vi "GetContextHelpInfo.vi"(0 "reference in":refnum<class "DQMHModuleNode.lvclass">, 1 "MousePos":T1 {"y" format="%.2f"; "x" format="%.2f"}, 5 "error in (no error)":errorcluster) -> (14 "reference out":refnum<class "DQMHModuleNode.lvclass">, 15 "ContextHelpInfoExist":bool, 16 "ContextHelpInfo":variant, 19 "error out":errorcluster)   [LabVIEW 2014, in "DQMHModuleNode.lvclass"]
doc: "GetContextHelpInfo"
uses:
  <resource>/Framework/Providers/Open_GDS/UML/DQMHModuleNode_class/DQMHModuleNode.lvclass
  <resource>/Framework/Providers/Open_GDS/UML/General/Point/Point Point2D.ctl
  <resource>/Framework/Providers/Open_GDS/UML/MultiLineString_class/MultiLineString.lvclass
  <resource>/Framework/Providers/Open_GDS/ClassProviders/Provider_BaseClassInterface/ClassReader_class/ClassReader.lvclass
  <resource>/Framework/Providers/Open_GDS/UML/RectangularNode_class/RectangularNode.lvclass
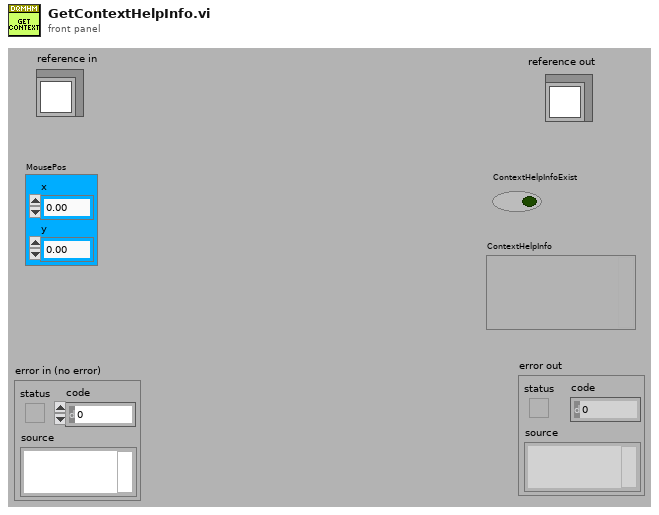
[diagram p1: front panel]
types:
  T1 = typedef "Point Point2D.ctl" = cluster{"x":dbl, "y":dbl}
  T2 = typedef "DQMHModuleNode.lvclass/ObjectAttributes.ctl" = cluster{"midHeight":dbl, "botHeight":dbl, "Name":refnum<class "MultiLineString.lvclass">, "Description":refnum<class "MultiLineString.lvclass">, "InternalData":refnum<class "MultiLineString.lvclass">, "Events":refnum<class "MultiLineString.lvclass">, "DEFAULT_COMPARTMENT_HEIGHT":i32, "DEFAULT_WIDTH":i32, "DEFAULT_HEIGHT":i32, "showEvents":bool, "showInternalData":bool, "ClassPath":path}
  T3 = typedef "RectangularNode.lvclass/ObjectAttributes.ctl" = cluster{"bounds":T4}
  T4 = typedef "Rectangle Rectangle2D.ctl" = cluster{"x":dbl, "y":dbl, "width":dbl, "height":dbl}
  T5 = cluster{"text":string, "empty picture":picture, "Description":string}
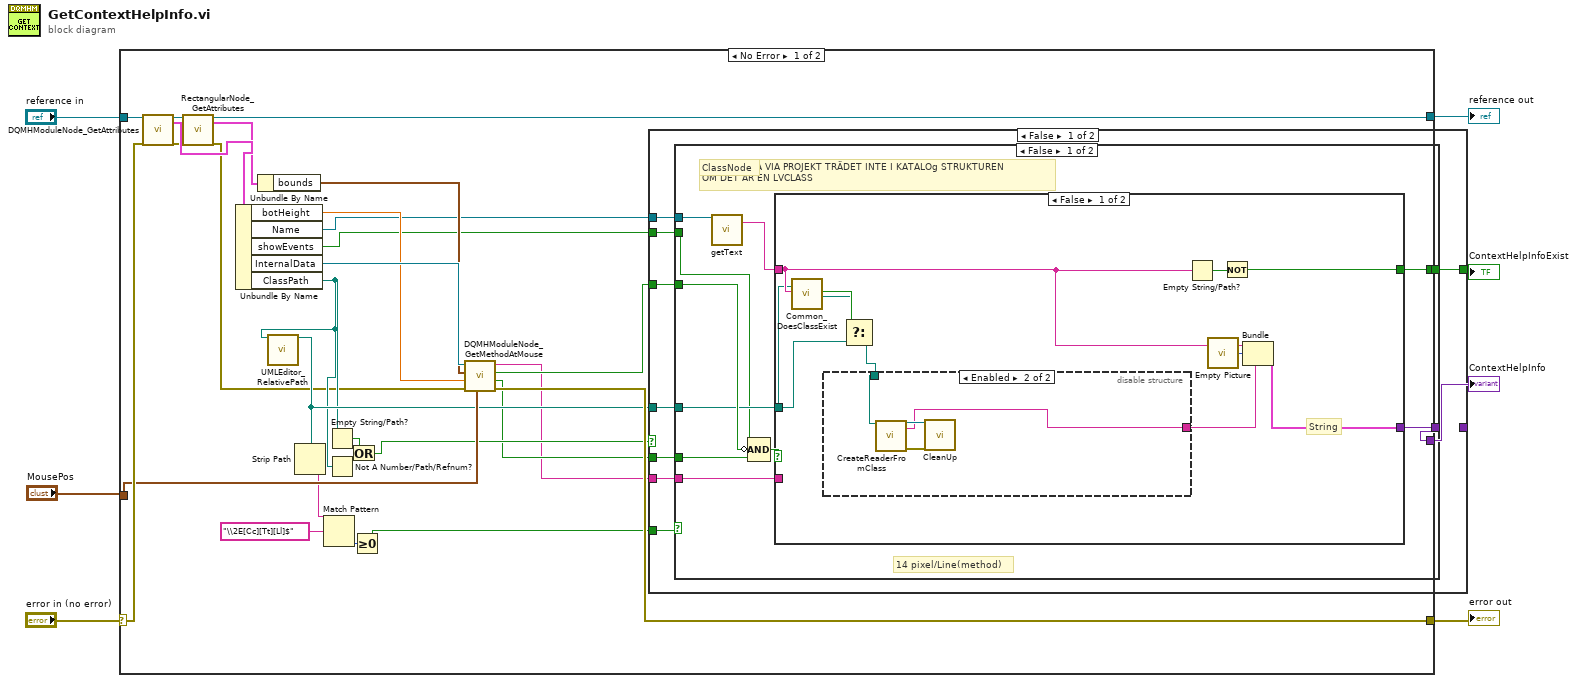
[diagram p0: block diagram]
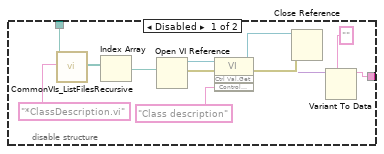
[diagram p2: hidden frame]
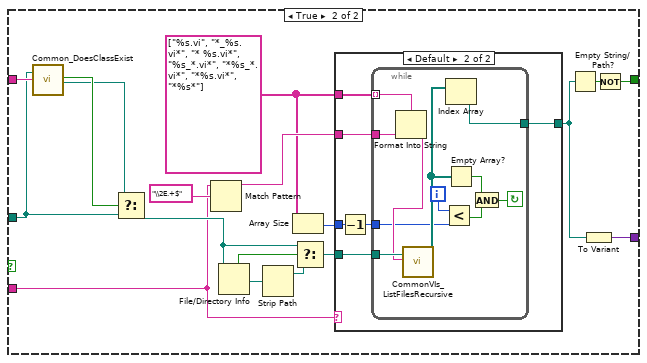
[diagram p3: hidden frame]
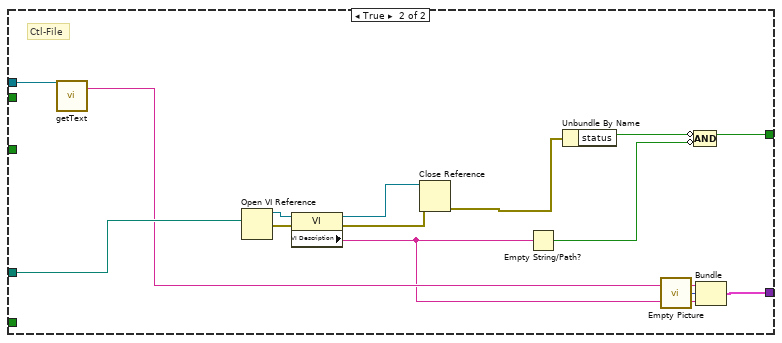
[diagram p5: hidden frame]
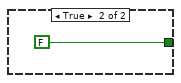
[diagram p6: hidden frame]
diagram:
  n1 = case shown="No Error" "error in (no error)" {
    selector: "error in (no error)" -> [w36 w132]
    tunnel: "reference in" -> [w35 w133]
    tunnel: [w32 w132] -> w5
    tunnel: [w9 w133] -> w4
    tunnel: "MousePos" -> [w33 _]
    tunnel: [w31 _] -> w2
    tunnel: [w30 _] -> w1
    frame No Error {
      n2 = call <resource>:"DQMHModuleNode_GetAttributes.vi"("reference in"=w35, "error in (no error)"=w36) -> ("reference out"=w12:refnum<class "DQMHModuleNode.lvclass">, "Data"=w13:T2, "error out"=w11:errorcluster)  [unwired: 1 in, 14 out]
      n3 = call <resource>:"RectangularNode_GetAttributes.vi"("reference in"=w12, "error in (no error)"=w11) -> ("reference out"=w9:refnum<class "DQMHModuleNode.lvclass">, "Data"=w8:T3, "error out"=w10:errorcluster)  [unwired: 14 in, 1 out]
      n4 = Unbundle By Name(w13) -> ("botHeight"=w28:dbl, "Name"=w25:refnum<class "MultiLineString.lvclass">, "showEvents"=w26:bool, "InternalData"=w34:refnum<class "MultiLineString.lvclass">, "ClassPath"=w16:path)
      n5 = Unbundle By Name(w8) -> ("bounds"=w29:T4)
      n6 = call <resource>:"UMLEditor_RelativePath.vi"("Path In"=w16) -> ("ConvertToAbsolutePath(If possible)"=w17:path)  [unwired: 1 in, 17 out]
      n7 = Strip Path(path=w17) -> (name=w21:string)  [unwired: 1 out]
      n8 = Match Pattern(string=w21, regular expression="\\2E[Cc][Tt][Ll]$") -> (offset past match=w19:i32)  [unwired: 4 out]
      n9 = Empty String/Path?(string/path=w16) -> (empty?=w24:bool)
      n10 = Not A Number/Path/Refnum?(number/path/refnum=w16) -> (NaN/Path/Refnum?=w23:bool)
      n11 = Or(x=w24, y=w23) -> (x .or. y?=w22:bool)
      n12 = Greater Or Equal To 0?(x=w19) -> (x >= 0?=w18:bool)
      n13 = call <resource>:"DQMHModuleNode_GetMethodAtMouse.vi"("MousePos"=w33, "error in"=w10, "botHeight"=w28, "bounds"=w29, "reference in"=w34) -> ("error out"=w32:errorcluster, "MethodSelected"=w15:bool, "NoMmethodsExists"=w27:bool, "MEthodName"=w14:string)  [unwired: 1 in]
      n14 = case shown="False" w22 {
        tunnel: [w45 _] -> w31
        tunnel: [w44 FALSE] -> w30
        tunnel: w27 -> [w43 _]
        tunnel: w26 -> [w41 _]
        tunnel: w25 -> [w40 _]
        tunnel: w17 -> [w42 _]
        tunnel: w18 -> [w39 _]
        tunnel: w15 -> [w38 _]
        tunnel: w14 -> [w37 _]
        frame False {
          n15 = case shown="False" w39 {
            tunnel: [w55 w120] -> w45
            tunnel: [w54 w122] -> w44
            tunnel: w43 -> [w52 _]
            tunnel: w42 -> [w51 w124]
            tunnel: w41 -> [w50 _]
            tunnel: w40 -> [w49 w119]
            tunnel: w38 -> [w47 _]
            tunnel: w37 -> [w46 _]
            frame False {
              # "MÅSTE SÖKA VIA PROJEKT TRÄDET INTE I KATALOg STRUKTUREN\nOM DET ÄR EN LVCLASS"
              # "ClassNode"
              # "14 pixel/Line(method)"
              n16 = call-dynamic "getText.vi"("reference"=w49) -> ("text"=w48:string)  [unwired: 1 in, 17 out]
              n17 = Compound Arithmetic op=AND(w50, invert w52, w47) -> (w53:bool)
              n18 = case shown="False" w53 {
                tunnel: w51 -> [w57 w96]
                tunnel: [w63 w98] -> w55
                tunnel: [w61 w91] -> w54
                tunnel: w48 -> [w58 w97]
                tunnel: w46 -> [_ w82]
                frame False {
                  # "String"
                  n19 = call <resource>:"Common_DoesClassExist.vi"("ClassPath"=w57, "ClassName"=w58) -> ("llb-class"=w60:bool, "llb/LvCLass-Path"=w59:path)  [unwired: 16 out]
                  n20 = Select(t=w59, s=w60, f=w57) -> (s? t:f=w56:path)
                  n21 = disable-structure shown="Enabled" {
                    disable-tunnel: [w67 w78] -> w64
                    disable-tunnel: w56 -> [w66 w79]
                    frame Disabled {
                      n22 = call <resource>:"CommonVIs_ListFilesRecursive.vi"("directory path"=w66, "FileSearchPattern"="*ClassDescription.vi") -> ("Files"=w77:path[])  [unwired: 14 in, 3 out]
                      n23 = Index Array(array=w77) -> (element=w75:path)  [unwired: 1 in]
                      n24 = Open VI Reference(vi path=w75) -> (vi reference=w73:refnum<vi>, error out=w74:errorcluster)  [unwired: 5 in]
                      n25 = invoke class="VI" method="Ctrl Val.Get"(reference=w73, error in=w74, "Control Name"="Class description") -> (reference out=w71:refnum<vi>, error out=w70:errorcluster, "Get Control Value Variant"=w69:variant)  [unwired: 1 in, 1 out]
                      n26 = Close Reference(reference=w71, error in (no error)=w70) -> ()  [unwired: 1 out]
                      n27 = Variant To Data(type="", Variant=w69) -> (data=w67:string)  [unwired: 1 in, 1 out]
                    }
                    frame Enabled {
                      n28 = call <resource>:"CreateReaderFromClass.vi"("ClassPath/LvClassRef"=w79) -> ("ClassReader"=w80:refnum<class "ClassReader.lvclass">, "Description"=w78:string, "error out"=w81:errorcluster)  [unwired: 1 in, 15 out]
                      n29 = call-dynamic "CleanUp.vi"("reference in"=w80, "error in (no error)"=w81) -> ()  [unwired: 18 out]
                    }
                  }
                  n30 = Empty String/Path?(string/path=w58) -> (empty?=w62:bool)
                  n31 = call "Empty Picture"() -> ("empty picture"=w65:picture)
                  n32 = Not(x=w62) -> (.not. x?=w61:bool)
                  n33 = Bundle("text"=w58, "empty picture"=w65, "Description"=w64) -> (w63:T5)  [unwired: 1 out]
                }
                frame True {
                  w87 = string[] ["%s.vi", "*_%s.vi*", "* %s.vi*", "%s_*.vi*", "*%s_*.vi*", "*%s.vi*", "*%s*"]
                  n34 = call <resource>:"Common_DoesClassExist.vi"("ClassPath"=w96, "ClassName"=w97) -> ("llb-class"=w95:bool, "llb/LvCLass-Path"=w94:path)  [unwired: 16 out]
                  n35 = Select(t=w94, s=w95, f=w96) -> (s? t:f=w83:path)
                  n36 = Match Pattern(string=w82, regular expression="\\2E.+$") -> (before substring=w88:string)  [unwired: 4 out]
                  n37 = File/Directory Info(path=w83) -> (path out=w85:path, directory=w90:bool)  [unwired: 1 in, 5 out]
                  n38 = Strip Path(path=w85) -> (stripped path=w84:path)  [unwired: 1 out]
                  n39 = Array Size(array=w87) -> (size(s)=w86:i32)
                  n40 = Select(t=w83, s=w90, f=w84) -> (s? t:f=w89:path)
                  n41 = case shown="Default" w82 {
                    tunnel: [_ w102] -> w93
                    tunnel: w89 -> [_ w105]
                    tunnel: w87 -> [_ w104]
                    tunnel: w88 -> [_ w103]
                    tunnel: w86 -> [_ w101]
                    frame "" {
                    }
                    frame Default {
                      n42 = Decrement(x=w101) -> (x-1=w100:i32)
                      n43 = while {
                        tunnel: w105 -> [w116]
                        tunnel: w104 -> [w115] mode=indexing
                        tunnel: w103 -> [w114]
                        tunnel: [w113] -> w102
                        tunnel: w100 -> [w109]
                        i -> [w110]
                        stop <- w106 continue-if-true
                        n44 = Format Into String(format string=w115, w114) -> (resulting string=w111:string)  [unwired: 2 in, 1 out]
                        n45 = call <resource>:"CommonVIs_ListFilesRecursive.vi"("directory path"=w116, "FileSearchPattern"=w111) -> ("Files"=w112:path[])  [unwired: 4 in, 13 out]
                        n46 = Less?(x=w110, y=w109) -> (x < y?=w107:bool)
                        n47 = Index Array(array=w112) -> (element=w113:path)  [unwired: 1 in]
                        n48 = Empty Array?(array=w112) -> (empty?=w108:bool)
                        n49 = And(x=w108, y=w107) -> (x .and. y?=w106:bool)
                      }
                    }
                  }
                  n50 = Empty String/Path?(string/path=w93) -> (empty?=w92:bool)
                  n51 = To Variant(anything=w93) -> (Variant=w98:variant)
                  n52 = Not(x=w92) -> (.not. x?=w91:bool)
                }
              }
            }
            frame True {
              # "Ctl-File"
              n53 = call-dynamic "getText.vi"("reference"=w119) -> ("text"=w118:string)  [unwired: 1 in, 17 out]
              n54 = Open VI Reference(vi path=w124) -> (vi reference=w129:refnum<vi>, error out=w130:errorcluster)  [unwired: 2 in, 3 out]
              n55 = property class="VI"(reference=w129, error in=w130) -> (reference out=w128:refnum<vi>, error out=w127:errorcluster, "VI Description"=w117:string)
              n56 = Close Reference(reference=w128, error in (no error)=w127) -> (error out=w126:errorcluster)
              n57 = Empty String/Path?(string/path=w117) -> (empty?=w123:bool)
              n58 = Unbundle By Name(w126) -> ("status"=w125:bool)
              n59 = call "Empty Picture"() -> ("empty picture"=w121:picture)
              n60 = Compound Arithmetic op=AND(invert w125, invert w123) -> (w122:bool)
              n61 = Bundle("text"=w118, "empty picture"=w121, "Description"=w117) -> (w120:T5)  [unwired: 1 out]
            }
          }
        }
        frame True {
        }
      }
    }
    frame Error {
    }
  }
  "reference out" <- w4
  "error out" <- w5
  "ContextHelpInfo" <- w2
  "ContextHelpInfoExist" <- w1
